vi "Thread@ForeachLoop__Parameter.vi"(1 "ParamterIn":string) -> (0 "ParamterOut":string)   [LabVIEW 2019]
uses:
  MainFrame/Global.vi
panel:
  in  "Variable":string(combo)
  in  "Thread Label":string(combo)
  in  "Confirm":bool
  # "Thread@ForeachLoop $Label,$Variable1(,Variable2......)\nEX:\nVariable@VariableSet Var1,[aaa;bbb;ccc;ddd]\nThread@ForeachStart Loop\nThread@ForeachLoop Loop, Var1"
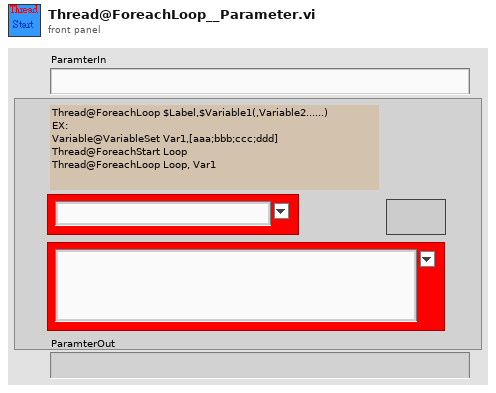
[diagram p1: front panel]
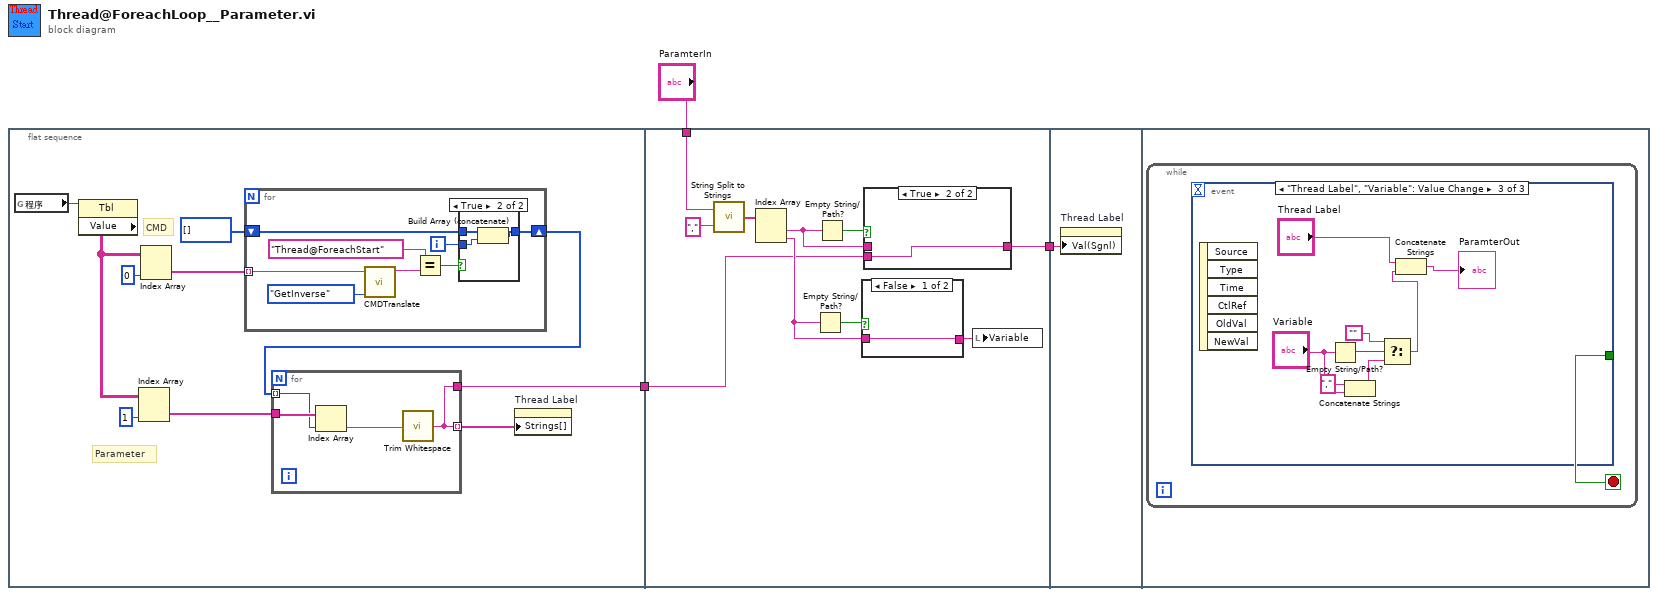
[diagram p0: block diagram]
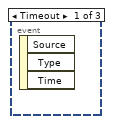
[diagram p5: hidden frame]
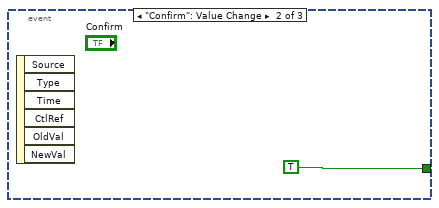
[diagram p6: hidden frame]
diagram:
  n1 = flat-sequence {
    tunnel: [w4] -> w1
    tunnel: "ParamterIn" -> [w37]
    tunnel: [w32] -> w2
    tunnel: w1 -> [w30]
    tunnel: w2 -> [w43]
    frame #0 {
      # "Parameter"
      # "CMD"
      n2 = global read "Global.vi" "程序"() -> (w13:refnum<vi>)
      n3 = property class="Tbl"(reference=w13) -> ("Value"=w10:string[][])  [unwired: 1 in, 2 out]
      n4 = Index Array(array=w10, index (col)=1 ("index (row)")) -> (element=w7:string[])  [unwired: 1 in]
      n5 = Index Array(array=w10, index (col)=0 ("index (row)")) -> (element=w9:string[])  [unwired: 1 in]
      n6 = for {
        tunnel: w9 -> [w24] mode=indexing
        shift-right: [w18] -> w6
        shift-left: i32[] [] -> [w20]
        i -> [w19]
        n7 = call "CMDTranslate.vi"("OP"=enum16{"Init", "Set", "Get", "GetInverse"}."GetInverse", "CMDIn"=w24) -> ("CMDOut"=w23:string)  [unwired: 9 in]
        n8 = Equal?(x="Thread@ForeachStart", y=w23) -> (x = y?=w21:bool)
        n9 = case shown="True" w21 {
          tunnel: w20 -> [w26 w29]
          tunnel: w19 -> [_ w28]
          tunnel: [w26 w27] -> w18
          frame False {
          }
          frame True {
            n10 = Build Array (concatenate)(w29, w28) -> (w27:i32[])
          }
        }
      }
      n11 = for {
        tunnel: w7 -> [w17]
        tunnel: w6 -> [w16] mode=indexing
        tunnel: [w15] -> w5 mode=indexing
        tunnel: [w15] -> w4
        n12 = Index Array(array=w17, index=w16) -> (element=w14:string)
        n13 = call <vilib>:"Trim Whitespace.vi"("string"=w14) -> ("trimmed string"=w15:string)  [unwired: 1 in]
      }
      n14 = property on="Thread Label" class="CmbBox"("Strings[]"=w5) -> ()  [unwired: 2 in, 2 out]
    }
    frame #1 {
      n15 = call "String Split to Strings.vi"("search string/char (-)"=",", "String"=w37) -> ("Array"=w39:string[])
      n16 = Index Array(array=w39) -> (element #1=w35:string, element #2=w33:string)  [unwired: 2 in]
      n17 = Empty String/Path?(string/path=w33) -> (empty?=w34:bool)
      n18 = Empty String/Path?(string/path=w35) -> (empty?=w36:bool)
      n19 = case shown="False" w34 {
        tunnel: w33 -> [w40 _]
        tunnel: [w40 _] -> w31
        frame False {
        }
        frame True {
        }
      }
      n20 = case shown="True" w36 {
        tunnel: w35 -> [w41 _]
        tunnel: [w41 w42] -> w32
        tunnel: w30 -> [_ w42]
        frame False {
        }
        frame True {
        }
      }
      n21 = local write "Variable"(w31) -> ()
    }
    frame #2 {
      n22 = property on="Thread Label" class="CmbBox"("Val(Sgnl)"=w43) -> ()  [unwired: 2 in, 2 out]
    }
    frame #3 {
      n23 = while {
        stop <- w44 stop-if-true
        n24 = event shown="[2] \"Thread Label\", \"Variable\": Value Change" {
          selector: _ -> [_ _ _]
          dyn-events: _ -> [_ _ _]
          timeout: _ -> [_ _ _]
          tunnel: [_ TRUE _] -> w44
          event Timeout {
            n25 = event-data() -> ()  [unwired: 1 in, 3 out]
          }
          event "Confirm": Value Change {
            n26 = event-data() -> ()  [unwired: 1 in, 6 out]
          }
          event "Thread Label", "Variable": Value Change {
            n27 = event-data() -> ()  [unwired: 1 in, 6 out]
            n28 = Empty String/Path?(string/path="Variable") -> (empty?=w52:bool)
            n29 = Concatenate Strings("," ("string"), "Variable") -> (w50:string)
            n30 = Select(t="", s=w52, f=w50) -> (s? t:f=w47:string)
            n31 = Concatenate Strings("Thread Label", w47) -> (→"ParamterOut":string)
          }
        }
      }
    }
  }
